vi "Clear-reference.vi"(8 "error in (no error)":errorcluster, 11 "Data ref.":refnum<data-value>) -> (0 "error out":errorcluster, 3 "Data":refnum<class "CV-Main.lvclass">)   [LabVIEW 2013, in "CameraVision.lvlib" / "CV-Main.lvclass"]
uses:
  CV-Main.lvclass
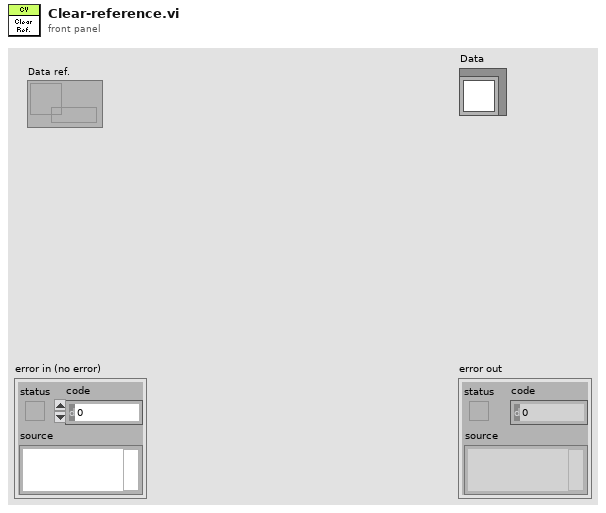
[diagram p1: front panel]
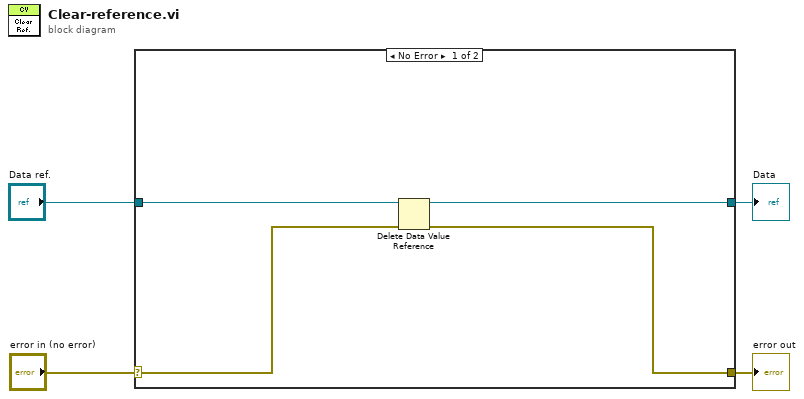
[diagram p0: block diagram]
diagram:
  n1 = case shown="No Error" "error in (no error)" {
    selector: "error in (no error)" -> [w7 w9]
    tunnel: [w5 w9] -> w3
    tunnel: [w6 _] -> w2
    tunnel: "Data ref." -> [w8 _]
    frame No Error {
      n2 = Delete Data Value Reference(data value reference=w8, error in=w7) -> (data value=w6:refnum<class "CV-Main.lvclass">, error out=w5:errorcluster)
    }
    frame Error {
    }
  }
  "error out" <- w3
  "Data" <- w2
